vi "zlgcan_demo_CANET.vi"() -> ()   [LabVIEW 2013]
doc: "适用的设备：CANET-E-U、CANET-2E-U、CANET-4E-U、CANET-8E-U、\nCANET-200T、CANET-100T"
uses:
  data_type/ZCAN_Transmit_Data.ctl
  data_type/ZCAN_InitCAN_setting_CANET.ctl
panel:
  in  "ZCAN_InitCAN_setting_CANET":T1
  in  "开启CAN":bool
  in  "stop":bool
  in  "?":T2(tab)
  in  "CAN卡型号":u32(ring)=4 items=["PCI5121"=1, "PCI9810"=2, "USBCAN-I"=3, "USBCAN-II"=4, "PCI9820"=5, "PCI5110"=7, "CANET-UDP"=12, "PCI9840B"=14, "PCI9820I"=16, "CANET-TCP"=17, "PCIE9221"=24, "PCI-5010-U"=19, "PCI-5020-U"=22, "USBCAN_E_U"=20, "USBCAN_2E_U"=21, "USBCAN-4E-U"=31, "USBCAN-8E-U"=34, "PCIE-CANFD-400U"=40, "PCIE-CANFD-200U"=39, "PCIE-CANFD-100U"=38, "USBCANFD-200U"=41, "USBCANFD-100U"=42, "USBCANFD-MINI"=43, "PCIE-9120I"=27, "PCIE-9110I"=28, "PCIE-9140I"=29, "CANDTU-MINI"=33, "CANDTU-200 XX"=32]
  in  "索引":u32(ring) items=["0", "1", "2", "3", "4", "5", "6", "7", "8"]
  in  "TCP模式":u32(ring) items=["客户端（client）", "服务器（server）"]
  in  "IP":string="192.168.0.178"
  in  "工作端口":u32=4001
  in  "本地端口":u32=6001
  out "设备句柄":u32
  out "通道句柄":u32
  out "error out":errorcluster caption="状态"
  in  "帧类型":u32(ring) items=["标准帧", "扩展帧"]
  in  "发送方式":u32(ring) items=["正常发送", "单次发送", "自发自收", "单次自发自收"]
  in  "帧格式":u32(ring) items=["数据帧", "远程帧"]
  out "数据长度":u8=8 max=8
  in  "ID":u32=18 format="0x%08x"
  in  "协议":u32(ring) items=["CAN"]
  in  "数据输入":string="11 22 33 44 55 66 77 88"
  in  "发送":bool
  in  "CAN数据帧数组":T3(array[cluster])
  out "CAN报文显示":string[][](table)
  in  "ZCAN_Transmit_Data":T4
  out "已接收帧数":u32
  # "适用的设备：CANET-E-U、CANET-2E-U、CANET-4E-U、CANET-8E-U、CANET-200T、CANET-100T"
  # "停止程序前，\n请先关闭CAN卡"
  # "当CANET的工作模式为：\n\n1. 客户端（TCP Client）\n\n   LabVIEW 设备型号选择【 CANET-TCP】\n\n   TCP模式选择【服务器 TCP Sever】\n\n   填写电脑本机IP+本地端口。\n\n2. 服务器（TCP Sever）\n\n   LabVIEW 设备型号选择【 CANET-TCP】\n\n   TCP模式选择【客户端 TCP Client】\n\n   填写CANET的 IP +工作端口\n\n3. UDP\n\n   LabVIEW 设备型号选择【 CANET-UDP】\n\n   填写CANET的IP+工作端口+本地端口"
  # "1. 调试运行DEMO前，将bin文件夹下面的kerneldlls文件夹先拷贝至LabView安装目录，\n如 D:\\Program Files (x86)\\National Instruments\\LabVIEW 2018。"
  # "2. 确保电脑有VC++ 2005/2008/2010/2013运行库（对应32，64位），可到微软官网下载。"
  # "3，如果打开设备失败，可能原因：\n（1）没有进行第二步操作；\n（2）已经打开过一次，没有正常关闭的情况下，继续点击“打开设备”，是无法打开的。\n     需要USB重新拔插，LABVIEW重启（全部关闭），然后再“打开设备”。\n (3) 项目路径不能有中文繁体。"
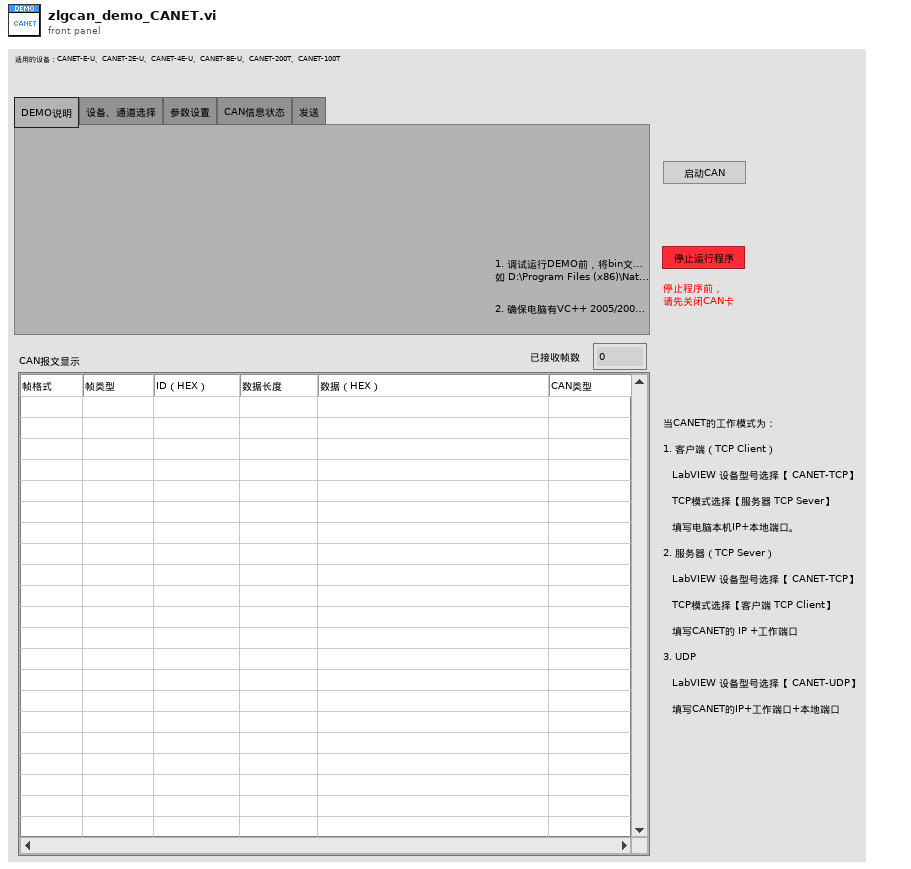
[diagram p1: front panel]
types:
  T1 = typedef "ZCAN_InitCAN_setting_CANET.ctl" = cluster{"tcp_type":u32, "work_port":u32, "local_port":u32, "IP":string}
  T2 = enum32{"DEMO说明", "设备、通道选择", "参数设置", "CAN信息状态", "发送"}
  T3 = cluster{u32, u8, u8, u8, u8, cluster{"[0]":u8, "[1]":u8, "[2]":u8, "[3]":u8, "[4]":u8, "[5]":u8, "[6]":u8, "[7]":u8}, u64}[]
  T4 = typedef "ZCAN_Transmit_Data.ctl" = cluster{"帧类型":u32, "帧格式":u32, "ID":u32, "数据长度":u8, "DATA":cluster{"CAN数据[0]":u8, "CAN数据[1]":u8, "CAN数据[2]":u8, "CAN数据[3]":u8, "CAN数据[4]":u8, "CAN数据[5]":u8, "CAN数据[6]":u8, "CAN数据[7]":u8}, "发送方式":u32}
  T5 = cluster{"[0]":u32, "[1]":u32, "[2]":u32, "[3]":u32, "[4]":u32, "[5]":u32, "[6]":u32, "[7]":u32}
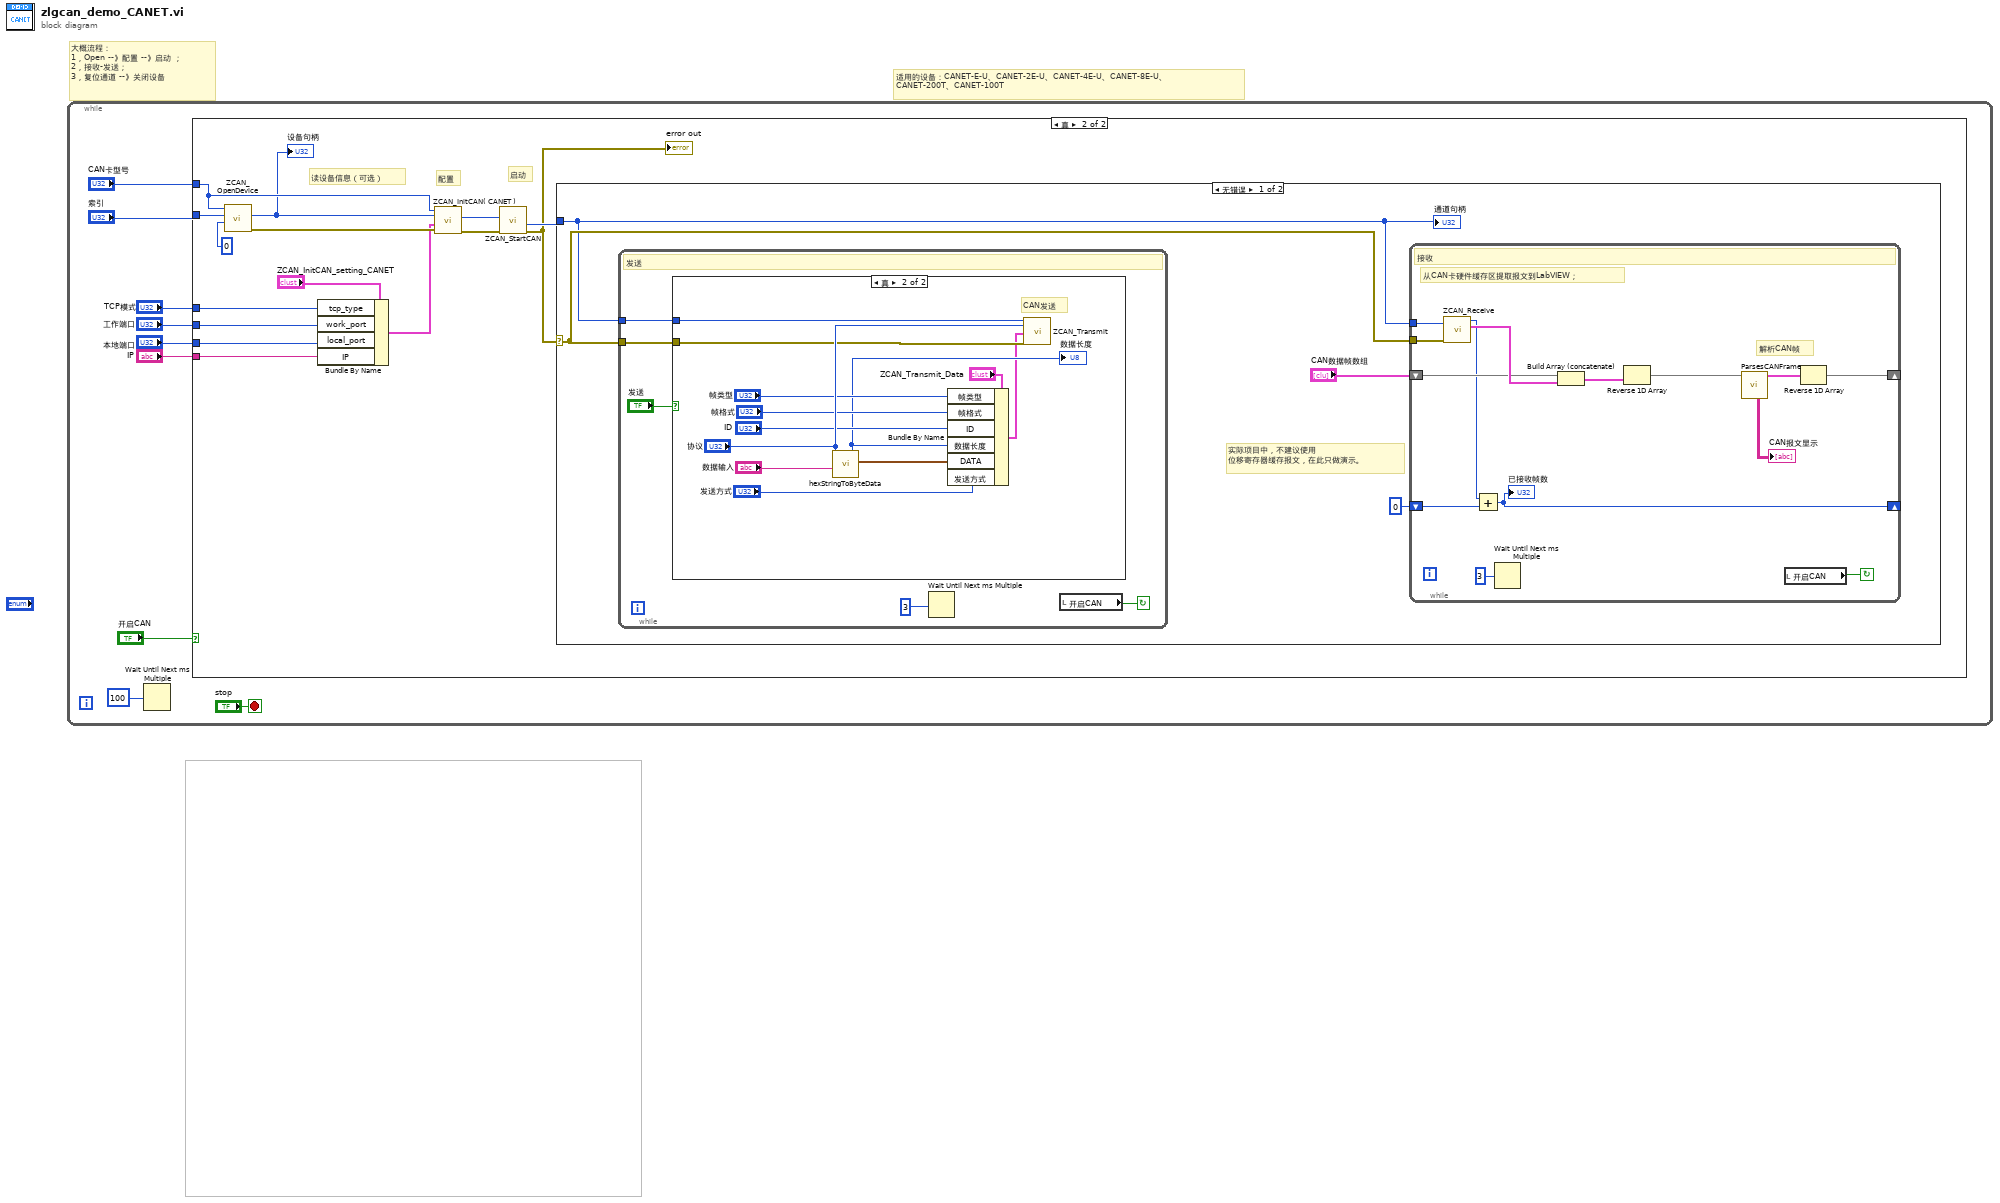
[diagram p0: block diagram]
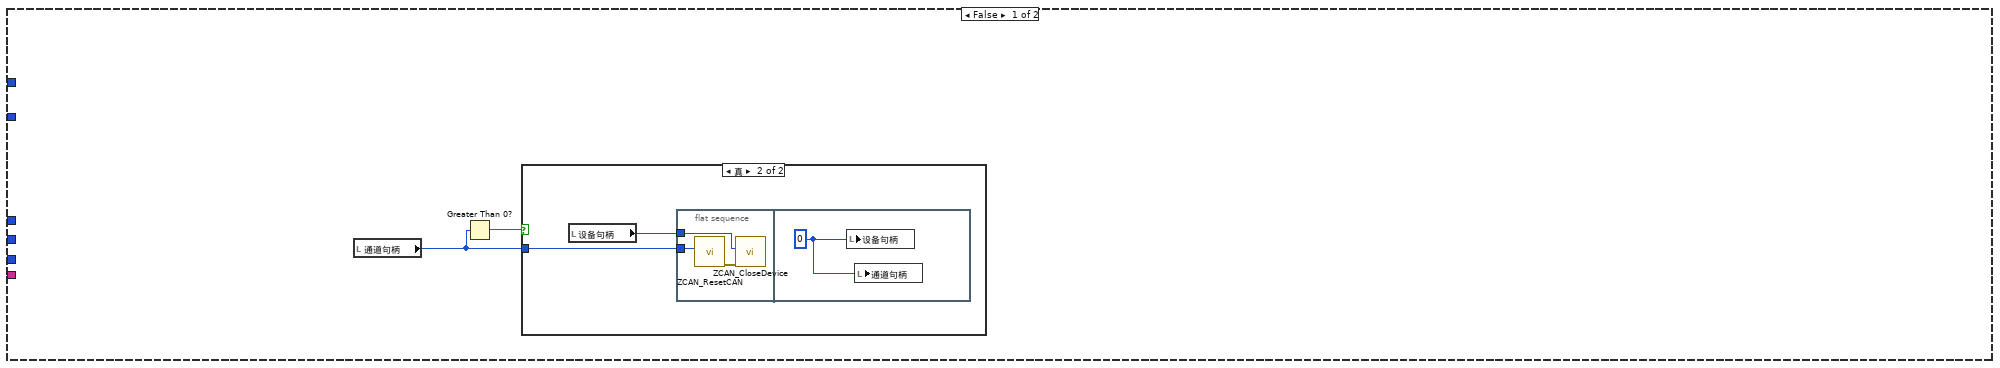
[diagram p2: hidden frame]
diagram:
  # "适用的设备：CANET-E-U、CANET-2E-U、CANET-4E-U、CANET-8E-U、\nCANET-200T、CANET-100T"
  # "大概流程：\n1，Open --》配置 --》启动 ；\n2，接收-发送；\n3，复位通道 --》关闭设备"
  n1 = while {
    stop <- "stop" stop-if-true
    n2 = Wait Until Next ms Multiple(millisecond multiple=u32 100) -> ()  [unwired: 1 out]
    n3 = case shown="真" "开启CAN" {
      tunnel: "CAN卡型号" -> [_ w27]
      tunnel: "索引" -> [_ w31]
      tunnel: "TCP模式" -> [_ w21]
      tunnel: "工作端口" -> [_ w20]
      tunnel: "本地端口" -> [_ w19]
      tunnel: "IP" -> [_ w18]
      frame False {
        # "关闭CAN卡"
        n4 = local read "通道句柄"() -> (w10:u32)
        n5 = Greater Than 0?(x=w10) -> (x > 0?=w11:bool)
        n6 = case shown="真" w11 {
          tunnel: w10 -> [_ w13]
          frame False {
          }
          frame True {
            n7 = local read "设备句柄"() -> (w12:u32)
            n8 = flat-sequence {
              tunnel: w13 -> [w15]
              tunnel: w12 -> [w14]
              frame #0 {
                n9 = call "ZCAN_ResetCAN.vi"("can_handle"=w15) -> ("error out"=w16:errorcluster)  [unwired: 9 in, 1 out]
                n10 = call "ZCAN_CloseDevice.vi"("error in (no error)"=w16, "device_handle"=w14) -> ()  [unwired: 8 in, 2 out]
              }
              frame #1 {
                w17 = u32 0 ("can_index_handle(out)")
                n11 = local write "设备句柄"(w17) -> ()
                n12 = local write "通道句柄"(w17) -> ()
              }
            }
          }
        }
      }
      frame True {
        # "启动"
        # "配置"
        # "读设备信息（可选）"
        n13 = call "ZCAN_OpenDevice.vi"("reserved"=0, "device_index"=w31, "device_type"=w27) -> ("error out"=w25:errorcluster, "DEVICE_HANDLE"=w26:u32)  [unwired: 7 in]
        "设备句柄" <- w26
        n14 = Bundle By Name(cluster="ZCAN_InitCAN_setting_CANET", "tcp_type"=w21, "work_port"=w20, "local_port"=w19, "IP"=w18) -> (w22:T1)
        n15 = call "ZCAN_InitCAN( CANET ).vi"("error in (no error)"=w25, "ZCAN_InitCAN_setting_CANET"=w22, "device_hande"=w26, "设备类型"=w27) -> ("error out"=w24:errorcluster, "can_index_handle"=w23:u32)  [unwired: 2 in]
        n16 = call "ZCAN_StartCAN.vi"("error in (no error)"=w24, "can_index_handle"=w23) -> ("error out"=w29:errorcluster, "can_index_handle(out)"=w30:u32)  [unwired: 7 in, 1 out]
        "error out" <- w29
        n17 = case shown="无错误" w29 {
          selector: w29 -> [w35 _]
          tunnel: w30 -> [w34 _]
          frame No Error {
            # "实际项目中，不建议使用\n位移寄存器缓存报文，在此只做演示。"
            n18 = while {
              tunnel: w34 -> [w53]
              tunnel: w35 -> [w51]
              stop <- w52 continue-if-true
              # "发送"
              n19 = case shown="真" "发送" {
                tunnel: w53 -> [_ w60]
                tunnel: w51 -> [_ w61]
                frame False {
                }
                frame True {
                  # "CAN发送"
                  n20 = call "hexStringToByteData.vi"("数据输入"="数据输入", "协议"="协议") -> ("CAN_data"=w57:T5, "字节数"=w62:i32)  [unwired: 7 in, 1 out]
                  "数据长度" <- w62
                  n21 = Bundle By Name(cluster="ZCAN_Transmit_Data", "帧类型"="帧类型", "帧格式"="帧格式", "ID"="ID", "数据长度"=w62, "DATA"=w57, "发送方式"="发送方式") -> (w56:T4)
                  n22 = call "ZCAN_Transmit.vi"("can_index_handle"=w60, "协议"="协议", "ZCAN_Transmit_Data"=w56, "error in (no error)"=w61) -> ()  [unwired: 15 in, 1 out]
                }
              }
              n23 = Wait Until Next ms Multiple(millisecond multiple=u32 3) -> ()  [unwired: 1 out]
              n24 = local read "开启CAN"() -> (w52:bool)
            }
            n25 = while {
              tunnel: w35 -> [w48]
              tunnel: w34 -> [w47]
              shift-right: [w49] -> _
              shift-left: 0 -> [w38]
              shift-right: [w41] -> _
              shift-left: "CAN数据帧数组" -> [w44]
              stop <- w46 continue-if-true
              # "从CAN卡硬件缓存区提取报文到LabVIEW；"
              # "解析CAN帧"
              # "接收"
              n26 = call "ZCAN_Receive.vi"("error in (no error)"=w48, "can_handle"=w47) -> ("CAN数据帧数组"=w45:T3, "Receive_Num"=w39:u32)  [unwired: 2 in, 2 out]
              n27 = Add(x=w39, y=w38) -> (x+y=w49:u32)
              "已接收帧数" <- w49
              n28 = Wait Until Next ms Multiple(millisecond multiple=u32 3) -> ()  [unwired: 1 out]
              n29 = Build Array (concatenate)(w44, w45) -> (w43:T3)
              n30 = Reverse 1D Array(array=w43) -> (reversed array=w40:T3)
              n31 = call "ParsesCANFrame.vi"("CAN数据帧数组"=w40) -> ("CAN数据帧数组(out)"=w42:T3, "CAN报文显示"=→"CAN报文显示":string[][])  [unwired: 9 in]
              n32 = local read "开启CAN"() -> (w46:bool)
              n33 = Reverse 1D Array(array=w42) -> (reversed array=w41:T3)
            }
            "通道句柄" <- w34
          }
          frame Error {
          }
        }
      }
    }
  }
